vi "Runner Tests.vi"(8 "error in (no error)":errorcluster) -> (0 "error out":errorcluster)   [LabVIEW 2013]
uses:
  classes/Test Runner/Test Runner.lvclass
  Unit Tests for Runner.lvclass
  classes/Test Runner.Folder/Test Runner.Folder.lvclass
  classes/Test Runner.Project/Test Runner.Project.lvclass
  classes/Test Runner.Collection/Test Runner.Collection.lvclass
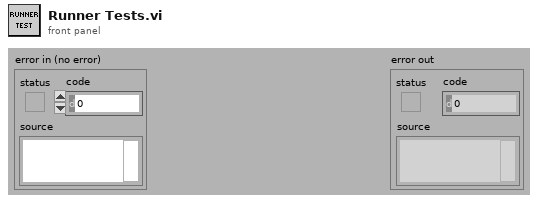
[diagram p1: front panel]
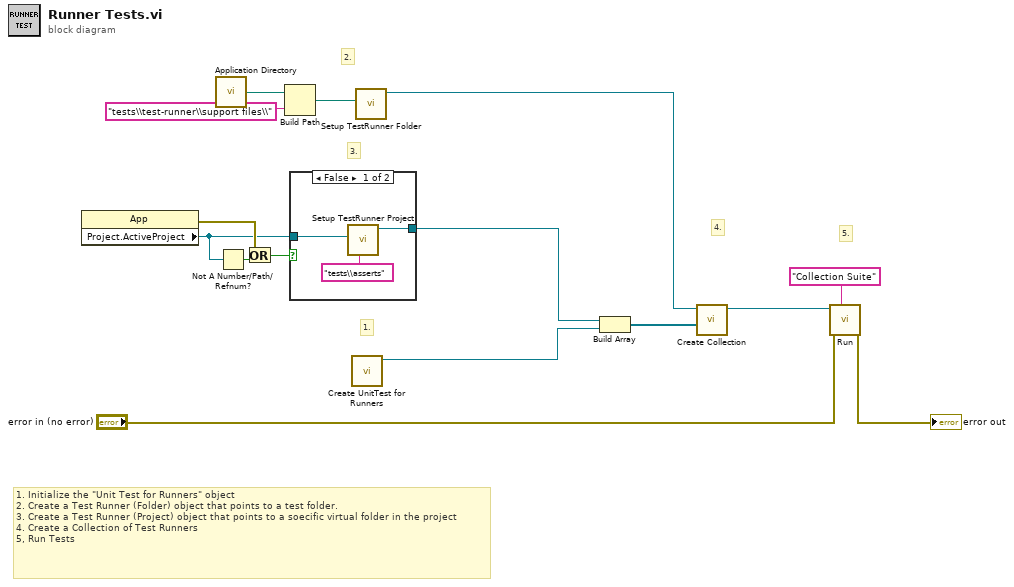
[diagram p0: block diagram]
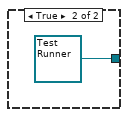
[diagram p2: hidden frame]
diagram:
  # "1."
  # "1. Initialize the \"Unit Test for Runners\" object\n2. Create a Test Runner (Folder) object that points to a test folder.\n3. Create a Test Runner (Project) object that points to a soecific virtual folder in the project\n4. Create a Collection of Test Runners\n5, Run Tests"
  # "5."
  # "4."
  # "3."
  # "2."
  n1 = property class="App"() -> (error out=w11:errorcluster, "Project.ActiveProject"=w10:refnum<vi>)  [unwired: 2 in, 1 out]
  n2 = call <vilib>:"Application Directory.vi"() -> ("Application Directory"=w15:path)
  n3 = Not A Number/Path/Refnum?(number/path/refnum=w10) -> (NaN/Path/Refnum?=w12:bool)
  n4 = Or(x=w11, y=w12) -> (x .or. y?=w9:bool)
  n5 = Build Path(base path=w15, name or relative path="tests\\test-runner\\support files\\") -> (appended path=w13:path)
  n6 = case shown="False" w9 {
    tunnel: [w18 refnum<class "Test Runner.lvclass"> refnum ("Caraya.lvlib:Test Runner.lvclass")] -> w1
    tunnel: w10 -> [w16 _]
    frame False {
      n7 = call "Setup TestRunner Project.vi"("Virtual Folder (empty: \"My Computer\")"="tests\\asserts" ("Virtual Folder (empty: \"My Computer\")"), "Project Refnum"=w16) -> ("Test Runner.Project out"=w18:refnum<class "Test Runner.Project.lvclass">)  [unwired: 8 in, 1 out]
    }
    frame True {
    }
  }
  n8 = call "Create UnitTest for Runners.vi"() -> ("Unit Tests for Runner out"=w3:refnum<class "Unit Tests for Runner.lvclass">)  [unwired: 10 in, 1 out]
  n9 = call "Setup TestRunner Folder.vi"("Directory to search"=w13) -> ("Test Runner.Folder out"=w4:refnum<class "Test Runner.Folder.lvclass">)  [unwired: 9 in, 1 out]
  n10 = Build Array(w1, w3) -> (w2:refnum<class "Test Runner.lvclass">[])
  n11 = call "Create Collection.vi"("Test Runners"=w2, "Test Runner 1"=w4) -> ("Test Runner.Collection out"=w5:refnum<class "Test Runner.Collection.lvclass">)  [unwired: 9 in]
  n12 = call "Run.vi"("Name"="Collection Suite", "error in (no error)"="error in (no error)", "Test Runner in"=w5) -> ("error out"=→"error out":errorcluster)  [unwired: 7 in, 1 out]
